vi "MEMR-Read Raw Data File.vi"(0 "Path":path=path "D:/Data/MEMR/Ken/SFMH41-MEMR-1.txt", 5 "Params":T1, 11 "error in":errorcluster) -> (8 "Array":dbl[][](array[numeric]), 15 "error out":errorcluster)   [LabVIEW 2020]
uses:
  Typedefs/MEMR-Params.ctl
  Typedefs/MEMR-Probe.ctl
  Typedefs/MEMR-Elicitor.ctl
  Human Studies/SFM Frontend/LV Source/Typedefs/HSTS-Transducer.ctl
  Typedefs/MEMR-Sequence.ctl
  Typedefs/MEMR-Analysis.ctl
  Typedefs/MEMR-Timing.ctl
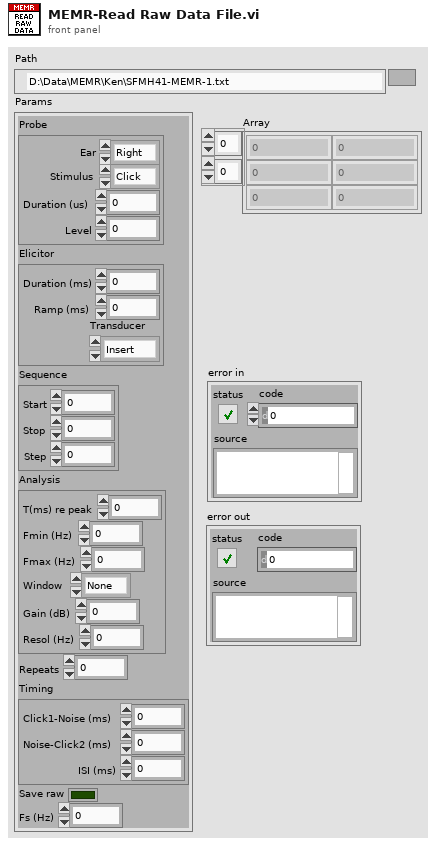
[diagram p1: front panel]
types:
  T1 = typedef "MEMR-Params.ctl" = cluster{"Probe":T2, "Elicitor":T3, "Sequence":T5, "Analysis":T6, "Repeats":i32, "Timing":T7, "Save raw":bool, "Fs (Hz)":dbl}
  T2 = typedef "MEMR-Probe.ctl" = cluster{"Ear":enum16{"Right", "Left"}, "Stimulus":enum16{"Click", "Chirp"}, "Duration (us)":dbl, "Level":dbl}
  T3 = typedef "MEMR-Elicitor.ctl" = cluster{"Duration (ms)":dbl, "Ramp (ms)":dbl, "Transducer":T4}
  T4 = typedef "HSTS-Transducer.ctl" = enum16{"Insert", "TDH-39", "HD300", "ER-10X"}
  T5 = typedef "MEMR-Sequence.ctl" = cluster{"Start":dbl, "Stop":dbl, "Step":dbl}
  T6 = typedef "MEMR-Analysis.ctl" = cluster{"T(ms) re peak":dbl, "Fmin (Hz)":dbl, "Fmax (Hz)":dbl, "Window":enum16{"None", "Hanning", "Hamming"}, "Gain (dB)":dbl, "Resol (Hz)":dbl}
  T7 = typedef "MEMR-Timing.ctl" = cluster{"Click1-Noise (ms)":dbl, "Noise-Click2 (ms)":dbl, "ISI (ms)":dbl}
  T8 = enum16{"open", "replace", "create", "open or create", "replace or create", "replace or create with confirmation"}
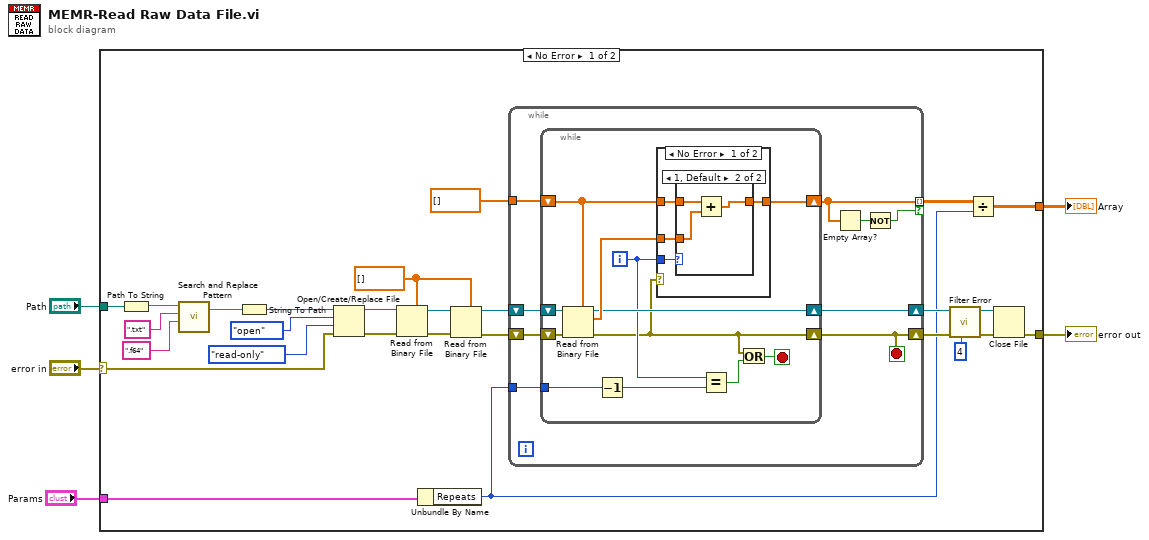
[diagram p0: block diagram]
diagram:
  n1 = case shown="No Error" "error in" {
    selector: "error in" -> [w10 w62]
    tunnel: "Path" -> [w13 _]
    tunnel: "Params" -> [w12 _]
    tunnel: [w9 w62] -> w2
    tunnel: [w7 _] -> w1
    frame No Error {
      w18 = dbl[] []
      n2 = Path To String(path=w13) -> (string=w31:string)
      n3 = call <vilib>:"Search and Replace Pattern.vi"("string"=w31, "regular expression (\"\")"=".txt" ("regular expression (\"\")"), "replace string (\"\")"=".f64" ("replace string (\"\")")) -> ("result string"=w28:string)  [unwired: 2 in, 1 out]
      n4 = String To Path(string=w28) -> (path=w27:path)
      n5 = Open/Create/Replace File(file path (use dialog)=w27, error in=w10, operation (0:open)=T8."open", access (0:read/write)=enum16{"read/write", "read-only", "write-only"}."read-only") -> (refnum out=w23:refnum<file>, error out=w24:errorcluster)  [unwired: 2 in, 1 out]
      n6 = Read from Binary File(5:w18, 8:w24, 11:w23) -> (0:w22:errorcluster, 3:w21:refnum<file>)  [unwired: 3 in, 2 out]
      n7 = Unbundle By Name(w12) -> ("Repeats"=w6:i32)
      n8 = Read from Binary File(5:w18, 8:w22, 11:w21) -> (0:w19:errorcluster, 3:w20:refnum<file>)  [unwired: 3 in, 2 out]
      n9 = while {
        tunnel: w6 -> [w37]
        shift-right: [w38] -> w17
        shift-left: w20 -> [w40]
        shift-right: [w35] -> w16
        shift-left: w19 -> [w39]
        tunnel: dbl[] [] -> [w36]
        tunnel: [w32] -> w8 mode=indexing if=w33
        stop <- w35 stop-if-true
        n10 = while {
          shift-right: [w48] -> w32
          shift-left: w36 -> [w49]
          shift-right: [w47] -> w38
          shift-left: w40 -> [w52]
          shift-right: [w43] -> w35
          shift-left: w39 -> [w51]
          tunnel: w37 -> [w46]
          i -> [w45]
          stop <- w42 stop-if-true
          n11 = Read from Binary File(5:w49, 8:w51, 11:w52) -> (0:w43:errorcluster, 2:w50:dbl[], 3:w47:refnum<file>)  [unwired: 3 in, 1 out]
          n12 = Decrement(x=w46) -> (x-1=w41:i32)
          n13 = case shown="No Error" w43 {
            tunnel: w50 -> [w56 _]
            tunnel: w49 -> [w55 w61]
            tunnel: [w54 w61] -> w48
            tunnel: w45 -> [w53 _]
            frame No Error {
              n14 = case shown="1, Default" w53 {
                tunnel: w56 -> [w57 w59]
                tunnel: w55 -> [_ w60]
                tunnel: [w57 w58] -> w54
                frame 0 {
                }
                frame 1, Default {
                  n15 = Add(x=w60, y=w59) -> (x+y=w58:dbl[])
                }
              }
            }
            frame Error {
            }
          }
          n16 = Equal?(x=w45, y=w41) -> (x = y?=w44:bool)
          n17 = Or(x=w43, y=w44) -> (x .or. y?=w42:bool)
        }
        n18 = Empty Array?(array=w32) -> (empty?=w34:bool)
        n19 = Not(x=w34) -> (.not. x?=w33:bool)
      }
      n20 = call "Filter Error.vi"("error in (no error)"=w16, "code to ignore"=4) -> ("error out"=w15:errorcluster)  [unwired: 9 in]
      n21 = Divide(x=w8, y=w6) -> (x/y=w7:dbl[][])
      n22 = Close File(refnum=w17, error in=w15) -> (error out=w9:errorcluster)  [unwired: 1 out]
    }
    frame Error {
    }
  }
  "error out" <- w2
  "Array" <- w1
